vi "电容充放电测试系统.vi"() -> ()   [LabVIEW 2024]
uses:
  <vilib>/Utility/file.llb/Write Delimited Spreadsheet (DBL).vi
  <vilib>/Utility/file.llb/Read Delimited Spreadsheet (DBL).vi
panel:
  out "充电状态":string
  out "电容电压":dbl
  out "放电时间":dbl
  out "充电时间":dbl
  in  "Vmax":dbl
  in  "C":dbl
  in  "R":dbl
  in  "选项卡控件":enum32{"实时波形图标显示", "充电波形", "放电波形"}(tab)
  out "波形图表":dbl(graph)
  in  "退出":bool
  in  "波形回放":bool
  in  "历史数据":bool
  in  "开始":bool
  # "RC模拟电路充放电性能测试"
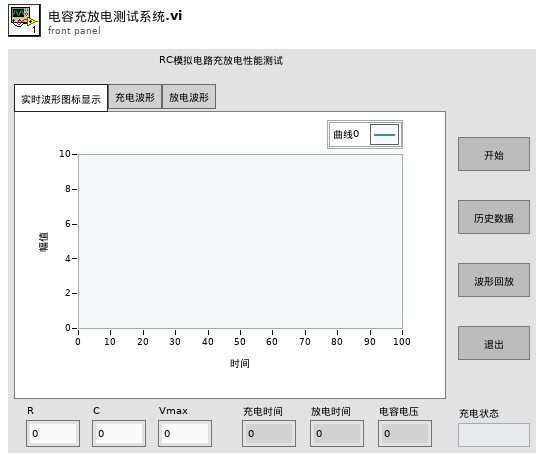
[diagram p1: front panel]
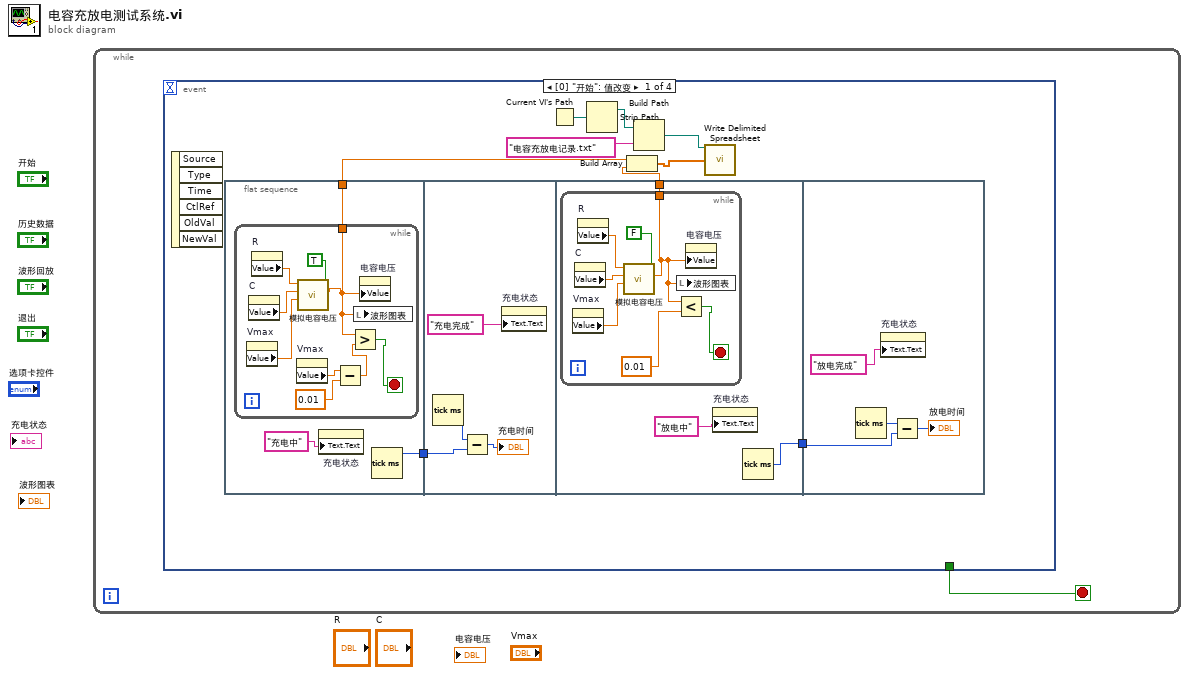
[diagram p0: block diagram]
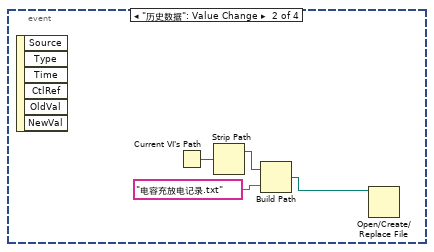
[diagram p2: hidden frame]
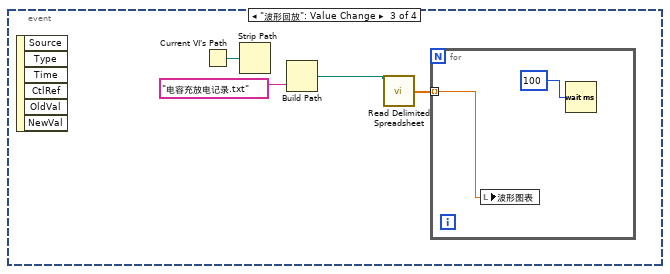
[diagram p3: hidden frame]
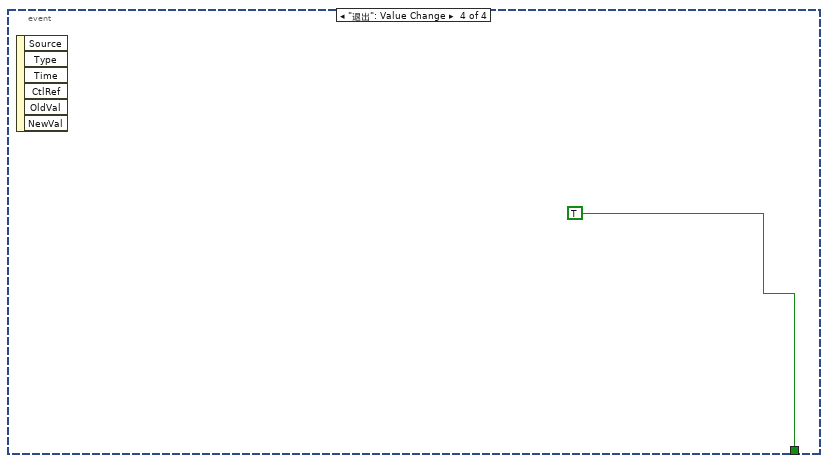
[diagram p4: hidden frame]
diagram:
  n1 = while {
    stop <- w1 stop-if-true
    n2 = event shown="[0] \"开始\": 值改变" {
      selector: _ -> [_ _ _ _]
      dyn-events: _ -> [_ _ _ _]
      timeout: _ -> [_ _ _ _]
      tunnel: [_ _ _ TRUE] -> w1
      event "开始": Value Change {
        n3 = event-data() -> ()  [unwired: 1 in, 6 out]
        n4 = flat-sequence {
          tunnel: [w13] -> w10
          tunnel: [w11] -> w4
          tunnel: w10 -> [w26]
          tunnel: [w29] -> w9
          tunnel: [w27] -> w3
          tunnel: w9 -> [w38]
          frame #0 {
            n5 = while {
              tunnel: [w14] -> w11
              stop <- w22 stop-if-true
              n6 = property on="Vmax" class="DigNum (严格)"() -> ("Value"=w19:dbl)  [unwired: 2 in, 2 out]
              n7 = property on="C" class="DigNum (严格)"() -> ("Value"=w20:dbl)  [unwired: 2 in, 2 out]
              n8 = property on="R" class="DigNum (严格)"() -> ("Value"=w21:dbl)  [unwired: 2 in, 2 out]
              n9 = property on="Vmax" class="DigNum (严格)"() -> ("Value"=w18:dbl)  [unwired: 2 in, 2 out]
              n10 = call "模拟电容电压.vi"("充电\n\n放电"=TRUE ("充电\n\n放电"), "Vmax"=w19, "C"=w20, "R"=w21) -> ("当前电压"=w14:dbl)  [unwired: 6 in, 1 out]
              n11 = Subtract(x=w18, y=0.01) -> (x-y=w17:dbl)
              n12 = Greater?(x=w14, y=w17) -> (0:w22:bool)
              n13 = local write "波形图表"(w14) -> ()
              n14 = property on="电容电压" class="DigNum (严格)"("Value"=w14) -> ()  [unwired: 2 in, 2 out]
            }
            n15 = property on="充电状态" class="Str"("Text.Text"="充电中" ("充电状态")) -> ()  [unwired: 2 in, 2 out]
            n16 = Tick Count (ms)() -> (millisecond timer value=w13:u32)
          }
          frame #1 {
            n17 = Tick Count (ms)() -> (millisecond timer value=w24:u32)
            n18 = Subtract(x=w24, y=w26) -> (x-y=→"充电时间":u32)
            n19 = property on="充电状态" class="Str"("Text.Text"="充电完成" ("f")) -> ()  [unwired: 2 in, 2 out]
          }
          frame #2 {
            n20 = while {
              tunnel: [w30] -> w27
              stop <- w36 stop-if-true
              n21 = property on="Vmax" class="DigNum (严格)"() -> ("Value"=w33:dbl)  [unwired: 2 in, 2 out]
              n22 = property on="C" class="DigNum (严格)"() -> ("Value"=w34:dbl)  [unwired: 2 in, 2 out]
              n23 = property on="R" class="DigNum (严格)"() -> ("Value"=w35:dbl)  [unwired: 2 in, 2 out]
              n24 = call "模拟电容电压.vi"("充电\n\n放电"=FALSE, "Vmax"=w33, "C"=w34, "R"=w35) -> ("当前电压"=w30:dbl)  [unwired: 6 in, 1 out]
              n25 = Less?(x=w30, y=0.01) -> (x < y?=w36:bool)
              n26 = local write "波形图表"(w30) -> ()
              n27 = property on="电容电压" class="DigNum (严格)"("Value"=w30) -> ()  [unwired: 2 in, 2 out]
            }
            n28 = property on="充电状态" class="Str"("Text.Text"="放电中" ("文本.文本")) -> ()  [unwired: 2 in, 2 out]
            n29 = Tick Count (ms)() -> (millisecond timer value=w29:u32)
          }
          frame #3 {
            n30 = Tick Count (ms)() -> (millisecond timer value=w39:u32)
            n31 = property on="充电状态" class="Str"("Text.Text"="放电完成" ("文本.文本")) -> ()  [unwired: 2 in, 2 out]
            n32 = Subtract(x=w39, y=w38) -> (x-y=→"放电时间":u32)
          }
        }
        n33 = Current VI's Path() -> (path=w6:path)
        n34 = Strip Path(path=w6) -> (stripped path=w7:path)  [unwired: 1 out]
        n35 = Build Array(w4, w3) -> (w2:dbl[])
        n36 = Build Path(base path=w7, name or relative path="电容充放电记录.txt") -> (appended path=w8:path)
        n37 = call-poly <vilib>:"Write Delimited Spreadsheet.vi"("file path (dialog if empty)"=w8, "1D data"=w2) -> ()  [unwired: 12 in, 2 out]
      }
      event "历史数据": Value Change {
        n38 = event-data() -> ()  [unwired: 1 in, 6 out]
        n39 = Current VI's Path() -> (path=w44:path)
        n40 = Strip Path(path=w44) -> (stripped path=w41:path)  [unwired: 1 out]
        n41 = Build Path(base path=w41, name or relative path="电容充放电记录.txt") -> (appended path=w42:path)
        n42 = Open/Create/Replace File(file path (use dialog)=w42) -> ()  [unwired: 5 in, 3 out]
      }
      event "波形回放": Value Change {
        n43 = event-data() -> ()  [unwired: 1 in, 6 out]
        n44 = Current VI's Path() -> (path=w48:path)
        n45 = Strip Path(path=w48) -> ()  [unwired: 2 out]
        n46 = Build Path(name or relative path="电容充放电记录.txt") -> (appended path=w45:path)  [unwired: 1 in]
        n47 = call-poly <vilib>:"Read Delimited Spreadsheet.vi"("file path (dialog if empty)"=w45) -> ("first row"=w46:dbl[])  [unwired: 9 in, 5 out]
        n48 = for {
          tunnel: w46 -> [w50] mode=indexing
          n49 = local write "波形图表"(w50) -> ()
          n50 = Wait (ms)(milliseconds to wait=u32 100 ("等待时间（毫秒）")) -> ()  [unwired: 1 out]
        }
      }
      event "退出": Value Change {
        n51 = event-data() -> ()  [unwired: 1 in, 6 out]
      }
    }
  }
